vi "OCV.vi"() -> ()   [LabVIEW 2020]
panel:
  out "OCV":dbl
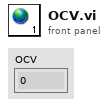
[diagram p1: front panel]
diagram:
